vi "UUT - initialize.vi"(8 "error in (no error)":errorcluster, 11 "VISA resource name":refnum<visa-resource-name>) -> (0 "error out":errorcluster, 3 "VISA resource name out":refnum<visa-resource-name>)   [LabVIEW 2011]
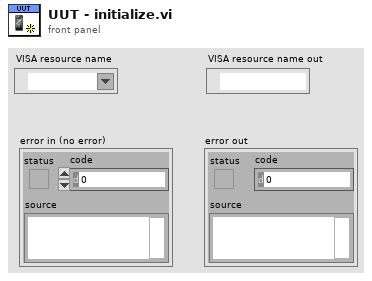
[diagram p1: front panel]
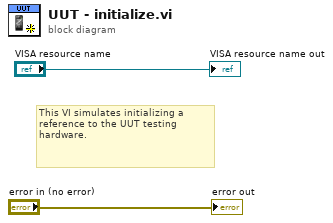
[diagram p0: block diagram]
diagram:
  # "This VI simulates initializing a reference to the UUT testing hardware."
  "error out" <- "error in (no error)"
  "VISA resource name out" <- "VISA resource name"
